vi "Teleop.vi"(10 "Match Info":T1={"Autonomous Elapsed Seconds"=0.0, "TeleOp Elapsed Seconds"=0.0, "Disabled Elapsed Seconds"=0.0, "Visited Autonomous"=FALSE, "Visited TeleOp"=FALSE, "Visited Disabled"=FALSE, "Autonomous Settings"={"Autonomous Style"=enum."Independent", "VI Refnum"=refnum}}, 11 "Call Context":T2) -> ()   [LabVIEW 2017]
doc: "This VI is called for each TeleOp packet received from the DS where the robot is not disabled. It is often used to read from the joysticks and update I/O or to update setpoints for timed control loops. It should complete and return within 20 milliseconds or it may miss DS packets."
uses:
  <vilib>/Rock Robotics/WPI/DriverStation/WPI_DriverStationDerivedRobotMode.ctl
  <vilib>/Rock Robotics/WPI/DriverStation/WPI_DriverStationMatch Info.ctl
  <vilib>/Rock Robotics/WPI/Solenoid/WPI_SolenoidValue.ctl
  <vilib>/Rock Robotics/WPI/Utilities/WPI_GetSetVariantRefNum.vi
  <vilib>/Rock Robotics/WPI/ThirdParty/Phoenix-LabVIEW/Motor Controller/Get/CTRE_Phoenix_MotorController_GetSelectedSensorData.vi
  <vilib>/Rock Robotics/Network Tables/NT Read Boolean.vi
  <vilib>/Rock Robotics/WPI/Joystick/WPI_JoystickArcadeMapping.vi
  <vilib>/Rock Robotics/Network Tables/NT Write Number.vi
panel:
  out "Brake is Enabled 6":bool
  out "Brake is Enabled 5":bool
  out "Brake is Enabled 4":bool
  out "Brake is Enabled 3":bool
  out "Brake is Enabled 2":bool
  out "Brake is Enabled":bool
  out "Shift Status":dbl
  # "DRIVER CONTROLS"
  # "This is the number that is multiplied with the joystick output to determine high \ngear turning speed, the lower the number the slower it will turn in high gear."
  # "These numbers controls overall how sensitive the joystick is to turning and foreward\nmovement, the lower the number is the faster it will respond to joystick motion. \nIf the number is 1 then it will move in a linear relationship with the joystick."
  # "This controls the maximum foreward and backwards speed of the robot, if at 1 then\nthe robot can move at max power, if at 0 then the robot cannot move at all."
  # "This turns the ability to use autoshift on/off, if activated it does NOT mean that \nautoshift is always on, it simply means that it can be turned on with buttons 6/11."
  # "This turns the ability to use high gear on/off, if activated it does NOT mean that \nhigh gear is always on, it simply means that it can be turned on with button 1."
  # "This turns on the ability to reverse the direction of the robot with the buttons 8/9."
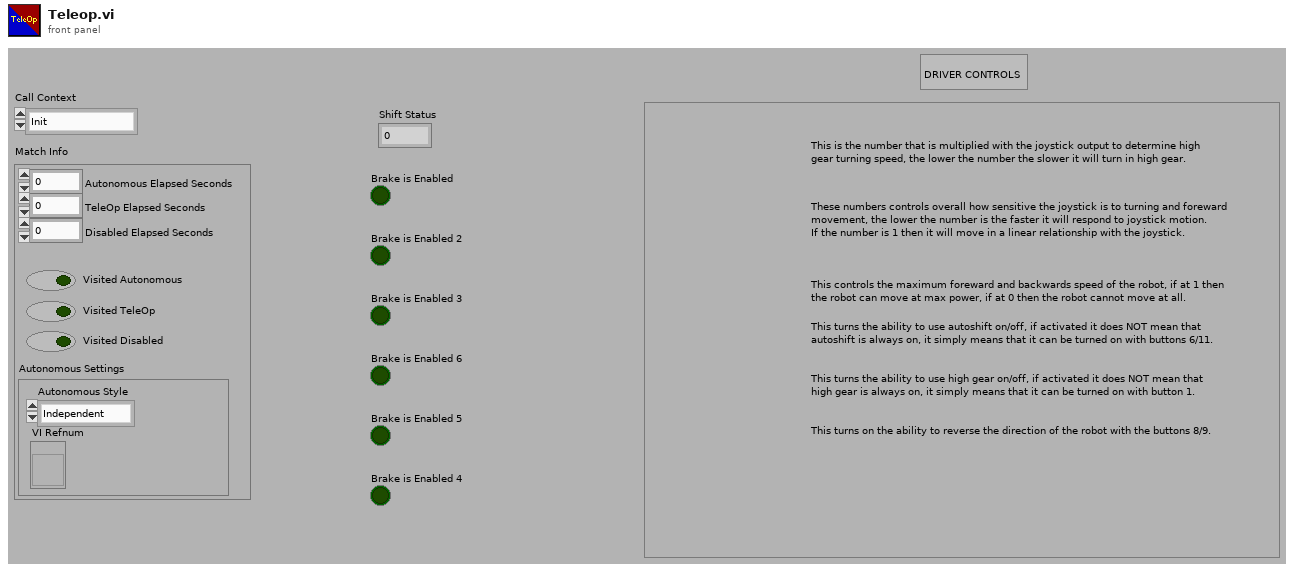
[diagram p1: front panel]
types:
  T1 = typedef "WPI_DriverStationMatch Info.ctl" = cluster{"Autonomous Elapsed Seconds":dbl, "TeleOp Elapsed Seconds":dbl, "Disabled Elapsed Seconds":dbl, "Visited Autonomous":bool, "Visited TeleOp":bool, "Visited Disabled":bool, "Autonomous Settings":cluster{"Autonomous Style":enum16{"Iterative", "Independent"}, "VI Refnum":refnum<vi>}}
  T2 = typedef "WPI_DriverStationDerivedRobotMode.ctl" = enum16{"Init", "Execute", "Stop"}
  T3 = typedef "WPI_JoystickDevRef.ctl" = cluster{"Device":T4}
  T4 = typedef "WPI_JoystickDeviceEnum.ctl" = enum16{"USB 0", "USB 1", "USB 2", "USB 3", "USB 4", "USB 5"}
  T5 = typedef "WPI_MotorControlDeviceRef.ctl" = cluster{"DeviceStatus":errorcluster, "Type":T6, "PWM":cluster{"PWM Channel":T7, "DeadBand":T8}, "CAN":cluster{"Device Number":u8, "SetOutput VI Ref":variant, "GetOutput VI Ref":variant, "Enable VI Ref":variant, "Disable VI Ref":variant, "Data":variant}, "Invert":bool, "DIO PWM":cluster{"PWM \"Enable\" Channel":T7, "DIOChannel":T9, "PWM Rate":dbl}}
  T6 = typedef "WPI_MotorControlType.ctl" = enum16{"PWM", "CAN", "DIO PWM"}
  T7 = typedef "FPGA_DIOPWMChannel.ctl" = enum8{"PWM 0", "PWM 1", "PWM 2", "PWM 3", "PWM 4", "PWM 5", "PWM 6", "PWM 7", "PWM 8", "PWM 9", "PWM MXP 0", "PWM MXP 1", "PWM MXP 2", "PWM MXP 3", "PWM MXP 4", "PWM MXP 5", "PWM MXP 6", "PWM MXP 7", "PWM MXP 8", "PWM MXP 9", "Invalid"}
  T8 = typedef "WPI_PWMDeadband.ctl" = cluster{"Name":string, "maxPositivePwm":i32, "minPositivePwm":i32, "centerPwm":i32, "maxNegativePwm":i32, "minNegativePwm":i32, "angularRange":u16}
  T9 = typedef "FPGA_DIOChannel.ctl" = enum8{"DIO 0", "DIO 1", "DIO 2", "DIO 3", "DIO 4", "DIO 5", "DIO 6", "DIO 7", "DIO 8", "DIO 9", "DIO MXP 0", "DIO MXP 1", "DIO MXP 2", "DIO MXP 3", "DIO MXP 4", "DIO MXP 5", "DIO MXP 6", "DIO MXP 7", "DIO MXP 8", "DIO MXP 9", "DIO MXP 10", "DIO MXP 11", "DIO MXP 12", "DIO MXP 13", "DIO MXP 14", "DIO MXP 15", "SPI Port CS1", "SPI Port CS2", "SPI Port CS3", "SPI Port MISO", "SPI Port MOSI", "Invalid"}
  T10 = typedef "WPI_SolenoidDevRef.ctl" = cluster{"DevStatus":errorcluster, "Pneumatics Control Module":u8, "Forward Solenoid Channel":T11, "Reverse Solenoid Channel":T11}
  T11 = typedef "WPI_SolenoidChannel.ctl" = enum8{"Solenoid 0", "Solenoid 1", "Solenoid 2", "Solenoid 3", "Solenoid 4", "Solenoid 5", "Solenoid 6", "Solenoid 7", "Invalid"}
  T12 = typedef "WPI_SolenoidValue.ctl" = enum16{"Off", "On", "Forward", "Reverse"}
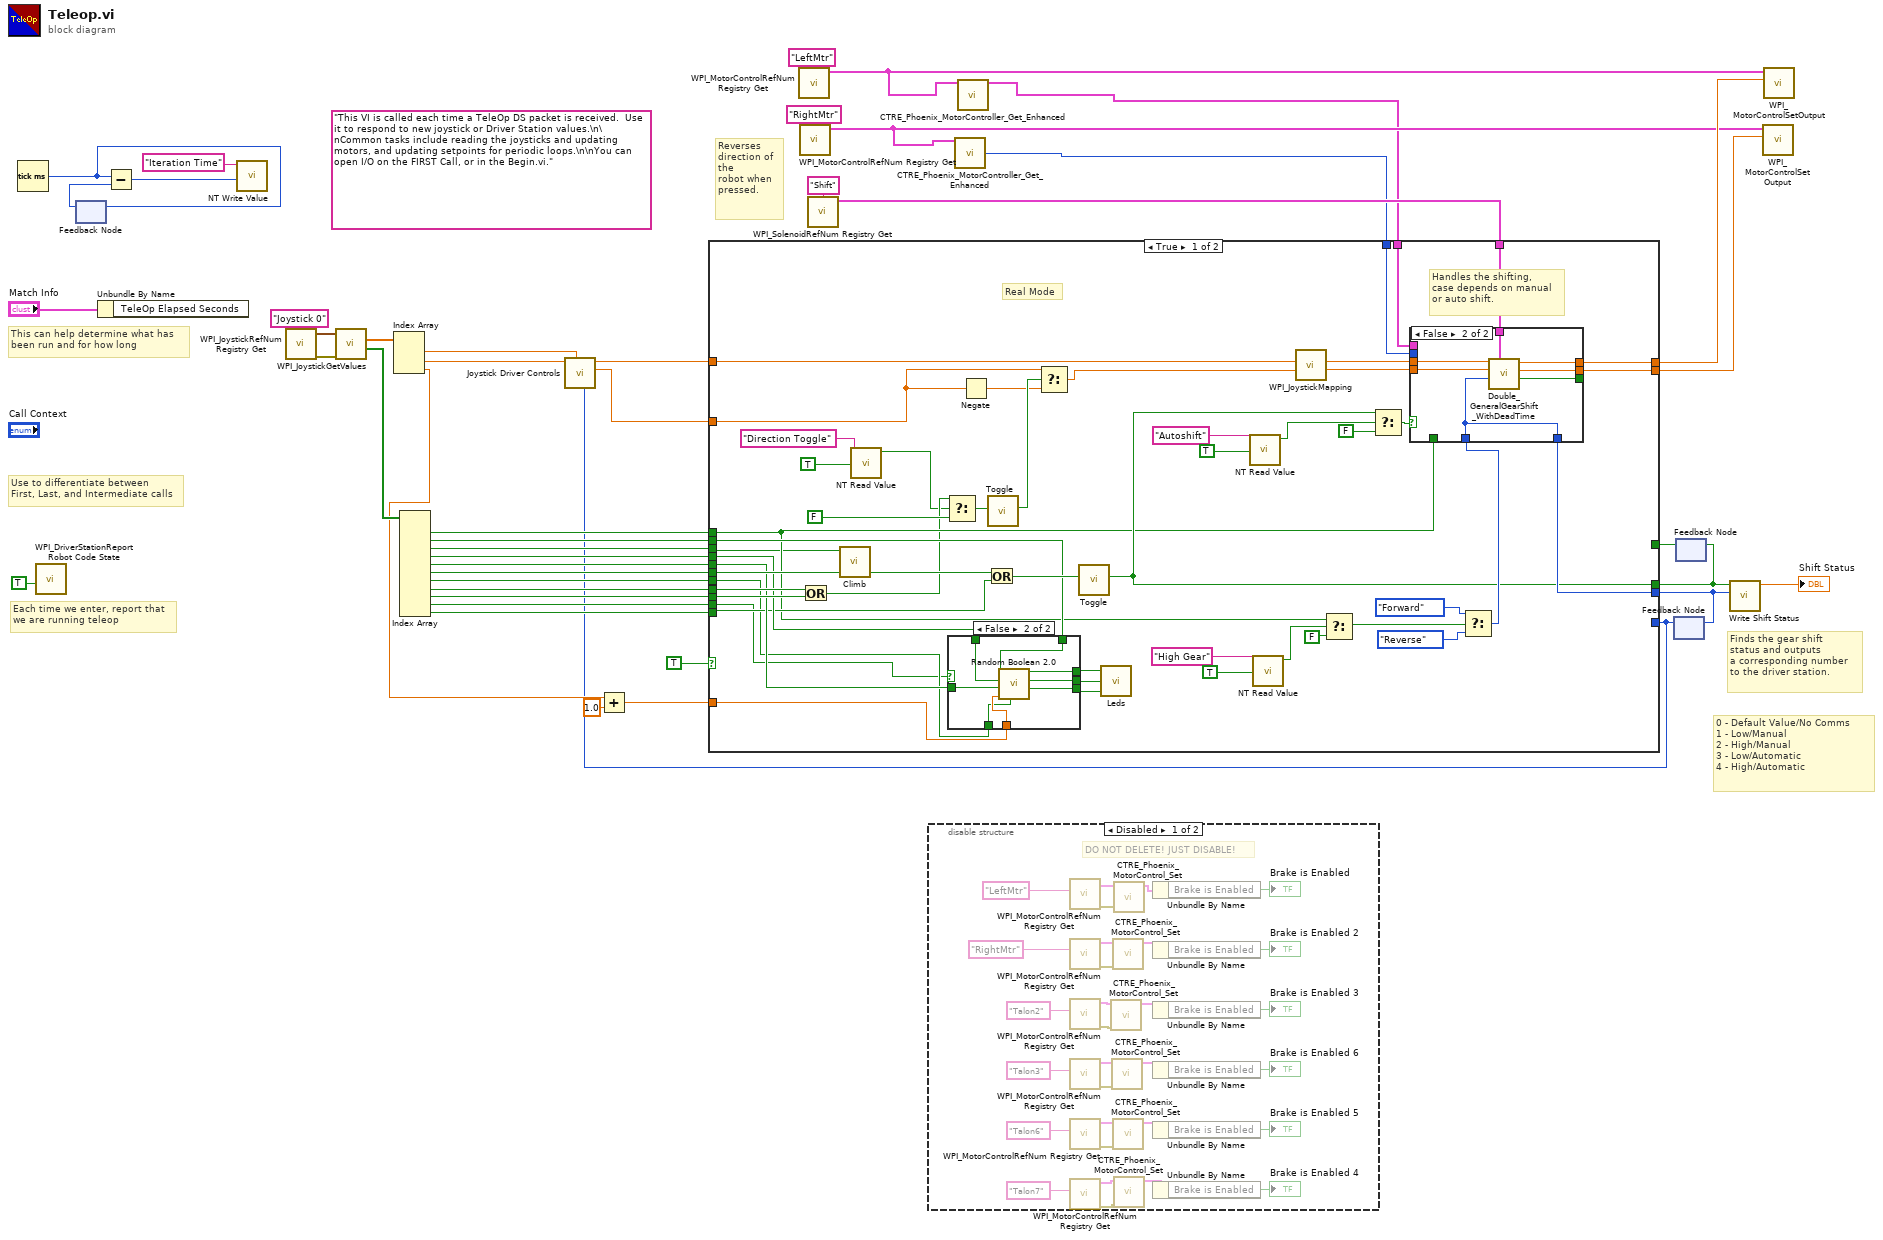
[diagram p0: block diagram]
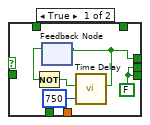
[diagram p2: hidden frame]
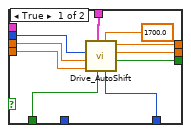
[diagram p3: hidden frame]
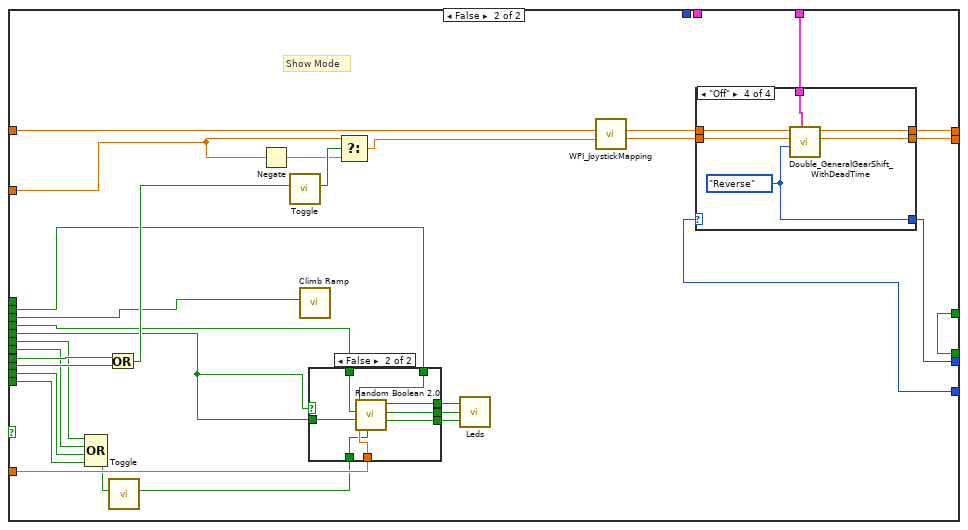
[diagram p4: hidden frame]
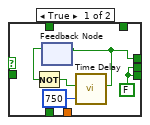
[diagram p5: hidden frame]
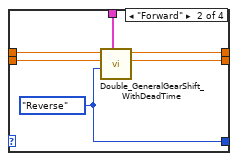
[diagram p7: hidden frame]
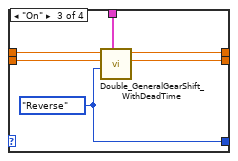
[diagram p8: hidden frame]
diagram:
  (unwired) "This VI is called each time a TeleOp DS packet is received.  Use it to respond to new joystick or Driver Station values.\n\nCommon tasks include reading the joysticks and updating motors, and updating setpoints for periodic loops.\n\nYou can open I/O on the FIRST Call, or in the Begin.vi."
  # "Reverses direction of the\nrobot when pressed."
  # "Finds the gear shift\nstatus and outputs\na corresponding number\nto the driver station."
  # "0 - Default Value/No Comms\n1 - Low/Manual\n2 - High/Manual\n3 - Low/Automatic\n4 - High/Automatic"
  # "Each time we enter, report that\nwe are running teleop"
  # "Use to differentiate between\nFirst, Last, and Intermediate calls"
  # "This can help determine what has\nbeen run and for how long"
  n1 = Tick Count (ms)() -> (millisecond timer value=w28:u32)
  n2 = call <vilib>:"WPI_DriverStationReport Robot Code State.vi"("TeleOp"=TRUE ("Autonomous")) -> ()  [unwired: 10 in, 1 out]
  n3 = feedback #1() -> (w29:u32)  [unwired: 1 in]
  n4 = feedback-in #1(w28) -> ()
  n5 = Unbundle By Name("Match Info") -> ()  [unwired: 1 out]
  n6 = Subtract(x=w28, y=w29) -> (x-y=w27:u32)
  n7 = call-poly <vilib>:"NT Write Value.vi"("Numeric"=w27, "Name"="Iteration Time") -> ()  [unwired: 9 in, 1 out]
  n8 = call <vilib>:"WPI_JoystickRefNum Registry Get.vi"("refnum name"="Joystick 0") -> ("error out"=w39:errorcluster, "JoystickDevRef"=w43:T3)  [unwired: 1 in, 8 out]
  n9 = call <vilib>:"WPI_JoystickGetValues.vi"("error in (no error)"=w39, "JoystickDevRef"=w43) -> ("Buttons"=w40:bool[], "Axes"=w41:dbl[])  [unwired: 5 in, 3 out]
  n10 = Index Array(array=w41) -> (element #1=w8:dbl, element #2=w7:dbl, element #3=w13:dbl)  [unwired: 3 in]
  n11 = Index Array(array=w40) -> (element #1=w20:bool, element #2=w16:bool, element #3=w21:bool, element #4=w15:bool, element #5=w14:bool, element #6=w34:bool, element #7=w35:bool, element #8=w37:bool, element #9=w38:bool, element #10=w23:bool, element #11=w22:bool)  [unwired: 11 in]
  n12 = Add(x=w13, y=1.0) -> (x+y=w12:dbl)
  n13 = call <vilib>:"WPI_MotorControlRefNum Registry Get.vi"("refnum name"="LeftMtr") -> ("MotorControlDevRef"=w2:T5)  [unwired: 9 in, 1 out]
  n14 = call <vilib>:"WPI_MotorControlRefNum Registry Get.vi"("refnum name"="RightMtr") -> ("MotorControlDevRef"=w4:T5)  [unwired: 9 in, 1 out]
  n15 = call <vilib>:"WPI_SolenoidRefNum Registry Get.vi"("refnum name"="Shift") -> ("SolenoidDevRef"=w33:T10)  [unwired: 9 in, 1 out]
  n16 = disable-structure shown="Disabled" {
    frame Disabled {
      # "DO NOT DELETE! JUST DISABLE!"
      n17 = call <vilib>:"WPI_MotorControlRefNum Registry Get.vi"("refnum name"="LeftMtr") -> ("error out"=w59:errorcluster, "MotorControlDevRef"=w58:T5)  [unwired: 9 in]
      n18 = call <vilib>:"WPI_MotorControlRefNum Registry Get.vi"("refnum name"="RightMtr") -> ("error out"=w61:errorcluster, "MotorControlDevRef"=w62:T5)  [unwired: 9 in]
      n19 = call <vilib>:"WPI_MotorControlRefNum Registry Get.vi"("refnum name"="Talon2") -> ("error out"=w64:errorcluster, "MotorControlDevRef"=w65:T5)  [unwired: 9 in]
      n20 = call <vilib>:"WPI_MotorControlRefNum Registry Get.vi"("refnum name"="Talon3") -> ("error out"=w67:errorcluster, "MotorControlDevRef"=w68:T5)  [unwired: 9 in]
      n21 = call <vilib>:"WPI_MotorControlRefNum Registry Get.vi"("refnum name"="Talon6") -> ("error out"=w71:errorcluster, "MotorControlDevRef"=w70:T5)  [unwired: 9 in]
      n22 = call <vilib>:"WPI_MotorControlRefNum Registry Get.vi"("refnum name"="Talon7") -> ("error out"=w74:errorcluster, "MotorControlDevRef"=w73:T5)  [unwired: 9 in]
      n23 = call <vilib>:"CTRE_Phoenix_MotorControl_Set.vi"("error in (no error)"=w64, "PhoenixMotorControlDevRef"=w65) -> ("PhoenixMotorControlDevRef"=w66:T5)  [unwired: 8 in, 1 out]
      n24 = call <vilib>:"CTRE_Phoenix_MotorControl_Set.vi"("error in (no error)"=w67, "PhoenixMotorControlDevRef"=w68) -> ("PhoenixMotorControlDevRef"=w69:T5)  [unwired: 8 in, 1 out]
      n25 = call <vilib>:"CTRE_Phoenix_MotorControl_Set.vi"("error in (no error)"=w61, "PhoenixMotorControlDevRef"=w62) -> ("PhoenixMotorControlDevRef"=w63:T5)  [unwired: 8 in, 1 out]
      n26 = call <vilib>:"CTRE_Phoenix_MotorControl_Set.vi"("error in (no error)"=w71, "PhoenixMotorControlDevRef"=w70) -> ("PhoenixMotorControlDevRef"=w72:T5)  [unwired: 8 in, 1 out]
      n27 = call <vilib>:"CTRE_Phoenix_MotorControl_Set.vi"("error in (no error)"=w59, "PhoenixMotorControlDevRef"=w58) -> ("PhoenixMotorControlDevRef"=w60:T5)  [unwired: 8 in, 1 out]
      n28 = call <vilib>:"CTRE_Phoenix_MotorControl_Set.vi"("error in (no error)"=w74, "PhoenixMotorControlDevRef"=w73) -> ("PhoenixMotorControlDevRef"=w75:T5)  [unwired: 8 in, 1 out]
      n29 = Unbundle By Name(w60) -> ("Brake is Enabled"=→"Brake is Enabled":bool)
      n30 = Unbundle By Name(w63) -> ("Brake is Enabled"=→"Brake is Enabled 2":bool)
      n31 = Unbundle By Name(w66) -> ("Brake is Enabled"=→"Brake is Enabled 3":bool)
      n32 = Unbundle By Name(w69) -> ("Brake is Enabled"=→"Brake is Enabled 6":bool)
      n33 = Unbundle By Name(w72) -> ("Brake is Enabled"=→"Brake is Enabled 5":bool)
      n34 = Unbundle By Name(w75) -> ("Brake is Enabled"=→"Brake is Enabled 4":bool)
    }
    frame Enabled {
    }
  }
  n35 = call-poly <vilib>:"CTRE_Phoenix_MotorController_Get_Enhanced.vi"("PhoenixMotorControlDevRef"=w4) -> ("Velocity (Raw Sensor Units per 100 ms)"=w3:i32)  [unwired: 11 in, 3 out]
  n36 = call-poly <vilib>:"CTRE_Phoenix_MotorController_Get_Enhanced.vi"("PhoenixMotorControlDevRef"=w2) -> ("PhoenixMotorControlDevRef"=w1:T5)  [unwired: 11 in, 3 out]
  n37 = feedback #2() -> (w10:T12)  [unwired: 1 in]
  n38 = call "Joystick Driver Controls.vi"("Shift Value"=w10, "X"=w8, "Y"=w7) -> ("Y"=w6:dbl, "X"=w9:dbl)  [unwired: 7 in]
  n39 = feedback #3() -> (w17:bool)  [unwired: 1 in]
  n40 = case shown="True" TRUE {
    tunnel: w38 -> [w124 w173]
    tunnel: w37 -> [w123 w172]
    tunnel: w35 -> [w97 w163]
    tunnel: w34 -> [w116 w164]
    tunnel: w33 -> [w115 w177]
    tunnel: w3 -> [w114 _]
    tunnel: [w113 w178] -> w32
    tunnel: [w112 w180] -> w30
    tunnel: w1 -> [w111 _]
    tunnel: [w110 w176] -> w19
    tunnel: w23 -> [w96 w162]
    tunnel: w22 -> [w98 w161]
    tunnel: w21 -> [w76 w155]
    tunnel: w20 -> [w89 _]
    tunnel: [w93 w175] -> w18
    tunnel: w9 -> [w107 w157]
    tunnel: w6 -> [w106 w156]
    tunnel: w10 -> [_ w174]
    tunnel: w17 -> [_ w175]
    tunnel: w16 -> [w101 w167]
    tunnel: w15 -> [w100 w169]
    tunnel: w14 -> [w99 w158]
    tunnel: w12 -> [w102 w165]
    frame True {
      # "Real Mode"
      # "Handles the shifting,\ncase depends on manual\nor auto shift."
      n41 = Or(x=w123, y=w124) -> (x .or. y?=w86:bool)
      n42 = call "Climb.vi"("Climb"=w76) -> ()  [unwired: 11 in]
      n43 = call-poly <vilib>:"NT Read Value.vi"("Default Value"=TRUE, "Name"="Direction Toggle") -> ("Boolean"=w77:bool)  [unwired: 8 in, 1 out]
      n44 = Select(t=w86, s=w77, f=FALSE) -> (s? t:f=w87:bool)
      n45 = case shown="False" w96 {
        tunnel: w99 -> [_ w136]
        tunnel: [w129 w131] -> w103
        tunnel: w100 -> [_ w135]
        tunnel: [w129 w132] -> w104
        tunnel: w101 -> [_ w134]
        tunnel: [w128 w133] -> w105
        tunnel: w102 -> [_ w137]
        tunnel: w97 -> [_ w130]
        frame True {
          w129 = FALSE
          n46 = feedback #4() -> (w127:bool)  [unwired: 1 in]
          n47 = Not(x=w127) -> (.not. x?=w126:bool)
          n48 = call "Time Delay.vi"("Time Delay"=u32 750, "Boolean in"=w126) -> ("Boolean out"=w128:bool)  [unwired: 9 in]
          n49 = feedback-in #4(w128) -> ()
        }
        frame False {
          n50 = call "Random Boolean 2.0.vi"("Output Random"=w130, "Cycle Time"=w137, "Boolean in 3"=w136, "Boolean in 2"=w135, "Boolean in 1"=w134) -> ("Boolean out 3"=w131:bool, "Boolean out 2"=w132:bool, "Boolean out 1"=w133:bool)  [unwired: 4 in]
        }
      }
      n51 = Negate(x=w106) -> (-x=w109:dbl)
      n52 = Or(x=w116, y=w98) -> (x .or. y?=w108:bool)
      n53 = call "Toggle.vi"("Input"=w87) -> ("Output"=w118:bool)  [unwired: 10 in]
      n54 = Select(t=w106, s=w118, f=w109) -> (s? t:f=w117:dbl)
      n55 = call "Toggle.vi"("Input"=w108) -> ("Output"=w93:bool)  [unwired: 10 in]
      n56 = call "Leds.vi"("R"=w103, "G"=w104, "B"=w105) -> ()  [unwired: 1 in]
      n57 = call-poly <vilib>:"NT Read Value.vi"("Default Value"=TRUE, "Name"="Autoshift") -> ("Boolean"=w80:bool)  [unwired: 8 in, 1 out]
      n58 = call-poly <vilib>:"NT Read Value.vi"("Default Value"=TRUE, "Name"="High Gear") -> ("Boolean"=w83:bool)  [unwired: 8 in, 1 out]
      n59 = call-poly <vilib>:"WPI_JoystickMapping.vi"("Y axis value"=w117, "X axis value"=w107) -> ("Right Motor Value"=w119:dbl, "Left Motor Value"=w120:dbl)  [unwired: 8 in]
      n60 = Select(t=w89, s=w83, f=FALSE) -> (s? t:f=w90:bool)
      n61 = Select(t=w93, s=w80, f=FALSE) -> (s? t:f=w94:bool)
      n62 = Select(t=WPI_SolenoidValue."Forward" ("Value"), s=w90, f=WPI_SolenoidValue."Reverse" ("Value")) -> (s? t:f=w95:T12)
      n63 = case shown="False" w94 {
        tunnel: [w145 w154] -> w112
        tunnel: [w146 w153] -> w113
        tunnel: w120 -> [w144 w152]
        tunnel: w119 -> [w143 w151]
        tunnel: w115 -> [w140 w149]
        tunnel: [w147 w150] -> _
        tunnel: w114 -> [w142 _]
        tunnel: w111 -> [_ _]
        tunnel: [w139 w148] -> w110
        tunnel: w95 -> [_ w148]
        tunnel: w89 -> [w138 _]
        frame True {
          n64 = call "Drive_AutoShift.vi"("Max"=1700.0, "Force Low Gear"=w138, "ShifterRef"=w140, "Right  Input"=w143, "Left Input"=w144, "Right RPM"=w142) -> ("Shifting"=w147:bool, "Right Output"=w146:dbl, "Left Output"=w145:dbl, "Gear"=w139:T12)  [unwired: 2 in]
        }
        frame False {
          n65 = call "Double_GeneralGearShift_WithDeadTime.vi"("ShifterRef"=w149, "Shift Value"=w148, "Right"=w151, "Left"=w152) -> ("Shifting"=w150:bool, "Right Output"=w153:dbl, "Left Output"=w154:dbl)  [unwired: 4 in, 1 out]
        }
      }
    }
    frame False {
      # "Show Mode"
      n66 = Compound Arithmetic op=OR(w164, w163, w162, w161) -> (w160:bool)
      n67 = Or(x=w172, y=w173) -> (x .or. y?=w171:bool)
      n68 = call "Toggle.vi"("Input"=w160) -> ("Output"=w159:bool)  [unwired: 10 in]
      n69 = Negate(x=w156) -> (-x=w182:dbl)
      n70 = call "Toggle.vi"("Input"=w171) -> ("Output"=w184:bool)  [unwired: 10 in]
      n71 = call "Climb Ramp.vi"("Climb"=w155) -> ()  [unwired: 11 in]
      n72 = case shown="False" w158 {
        tunnel: w158 -> [_ w197]
        tunnel: [w189 w196] -> w170
        tunnel: w169 -> [_ w195]
        tunnel: [w189 w194] -> w168
        tunnel: w167 -> [_ w193]
        tunnel: [w188 w192] -> w166
        tunnel: w165 -> [_ w191]
        tunnel: w159 -> [_ w190]
        frame True {
          w189 = FALSE
          n73 = feedback #5() -> (w187:bool)  [unwired: 1 in]
          n74 = Not(x=w187) -> (.not. x?=w186:bool)
          n75 = call "Time Delay.vi"("Time Delay"=u32 750, "Boolean in"=w186) -> ("Boolean out"=w188:bool)  [unwired: 9 in]
          n76 = feedback-in #5(w188) -> ()
        }
        frame False {
          n77 = call "Random Boolean 2.0.vi"("Output Random"=w190, "Cycle Time"=w191, "Boolean in 3"=w197, "Boolean in 2"=w195, "Boolean in 1"=w193) -> ("Boolean out 3"=w196:bool, "Boolean out 2"=w194:bool, "Boolean out 1"=w192:bool)  [unwired: 4 in]
        }
      }
      n78 = Select(t=w156, s=w184, f=w182) -> (s? t:f=w183:dbl)
      n79 = call "Leds.vi"("R"=w170, "G"=w168, "B"=w166) -> ()  [unwired: 1 in]
      n80 = call-poly <vilib>:"WPI_JoystickMapping.vi"("Y axis value"=w183, "X axis value"=w157) -> ("Right Motor Value"=w179:dbl, "Left Motor Value"=w181:dbl)  [unwired: 8 in]
      n81 = case shown="\"Off\"" w174 {
        selector: w174 -> [w198 _ _ _]
        tunnel: [w200 w203 w209 w215] -> w180
        tunnel: w181 -> [w200 w205 w211 w217]
        tunnel: w179 -> [w199 w204 w210 w216]
        tunnel: [w199 w202 w208 w214] -> w178
        tunnel: w177 -> [_ w206 w212 w218]
        tunnel: [w198 w201 w207 w213] -> w176
        frame "Reverse", Default {
        }
        frame "Forward" {
          w201 = WPI_SolenoidValue."Reverse" ("Shift Value")
          n82 = call "Double_GeneralGearShift_WithDeadTime.vi"("ShifterRef"=w206, "Shift Value"=w201, "Right"=w204, "Left"=w205) -> ("Right Output"=w202:dbl, "Left Output"=w203:dbl)  [unwired: 4 in, 2 out]
        }
        frame "On" {
          w207 = WPI_SolenoidValue."Reverse" ("Shift Value")
          n83 = call "Double_GeneralGearShift_WithDeadTime.vi"("ShifterRef"=w212, "Shift Value"=w207, "Right"=w210, "Left"=w211) -> ("Right Output"=w208:dbl, "Left Output"=w209:dbl)  [unwired: 4 in, 2 out]
        }
        frame "Off" {
          w213 = WPI_SolenoidValue."Reverse" ("Shift Value")
          n84 = call "Double_GeneralGearShift_WithDeadTime.vi"("ShifterRef"=w218, "Shift Value"=w213, "Right"=w216, "Left"=w217) -> ("Right Output"=w214:dbl, "Left Output"=w215:dbl)  [unwired: 4 in, 2 out]
        }
      }
    }
  }
  n85 = feedback-in #2(w19) -> ()
  n86 = feedback-in #3(w18) -> ()
  n87 = call "Write Shift Status.vi"("Gear"=w19, "Output"=w18) -> ("Shift Status"=→"Shift Status":dbl)  [unwired: 9 in]
  n88 = call <vilib>:"WPI_MotorControlSetOutput.vi"("Output"=w32, "MotorControlDevRef"=w4) -> ()  [unwired: 7 in, 3 out]
  n89 = call <vilib>:"WPI_MotorControlSetOutput.vi"("Output"=w30, "MotorControlDevRef"=w2) -> ()  [unwired: 7 in, 3 out]
